vi "GEA2 Send Message.vi"(0 "GEA2 Reference In":refnum<k24>, 1 "Input Data":T1 {"Command" format="%02x"; "Destination" format="%02x"; "Source" format="%02x"}, 2 "Retry Count":u32=3, 11 "Error In":errorcluster) -> (4 "GEA2 Reference Out":refnum<k24>, 15 "Error Out":errorcluster)   [LabVIEW 2014, in "GEA2_Toolkit.lvlib"]
doc: "This VI sends a GEA2 message accross the GEA2 bus."
uses:
  library/GEA2_Toolkit.lvlib
  C:/Automation/DLLs/PC Tools .NET/GeaCommunication.dll
  Automation/DLLs/PC Tools .NET/GeaCommunication.dll
  type defs/Data In.ctl
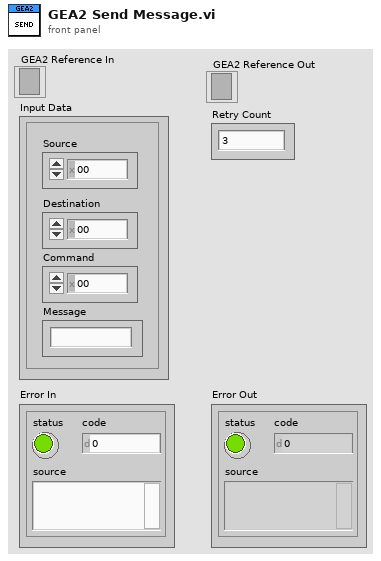
[diagram p1: front panel]
types:
  T1 = typedef "GEA2_Toolkit.lvlib/Data In.ctl" = cluster{"Source":u8, "Destination":u8, "Command":u8, "Message":string}
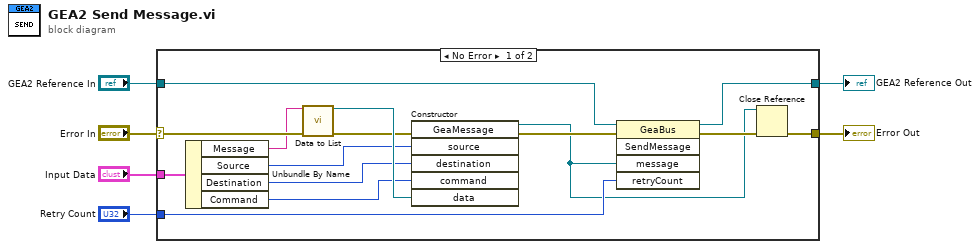
[diagram p0: block diagram]
diagram:
  n1 = case shown="No Error" "Error In" {
    selector: "Error In" -> [w18 w22]
    tunnel: "GEA2 Reference In" -> [w17 w23]
    tunnel: [w16 w23] -> w3
    tunnel: [w12 w22] -> w5
    tunnel: "Retry Count" -> [w15 _]
    tunnel: "Input Data" -> [w11 _]
    frame No Error {
      n2 = Unbundle By Name(w11) -> ("Message"=w9:string, "Source"=w10:u8, "Destination"=w8:u8, "Command"=w7:u8)
      n3 = call "Data to List.vi"("Data String In"=w9, "error in"=w18) -> ("Data List Out"=w20:refnum<k24>, "error out"=w19:errorcluster)  [unwired: 12 in]
      n4 = constructor class="GeaMessage"(error in=w19, "source"=w10, "destination"=w8, "command"=w7, "data"=w20) -> (reference out=w13:refnum<k24>, error out=w21:errorcluster)  [unwired: 2 in, 5 out]
      n5 = invoke class="GeaBus" method="SendMessage"(reference=w17, error in=w21, "message"=w13, "retryCount"=w15) -> (reference out=w16:refnum<k24>, error out=w14:errorcluster)  [unwired: 1 in, 3 out]
      n6 = Close Reference(reference=w13, error in (no error)=w14) -> (error out=w12:errorcluster)
    }
    frame Error {
    }
  }
  "Error Out" <- w5
  "GEA2 Reference Out" <- w3
